vi "Write to the File.vi"(7 "Data Cluster In":T1={"UI Reference"={"All Ctrl's Label's"=[], "ChannelListTree"=refnum, "All Object Ref"=[]}, "Tree Selection"={"Selected Channel"="", "Selected Interface"="", "Selected HW"="", "Tree Root Name"="", "Selected Module"=""}, "Selected File Path"=path "", "Selected HW"={"Slctd Hw Name"=[], "Slctd HW IP"=[]}, "Channel Config Path"=path "", "Interface Data"={"DO Channel's"=[]}, "General Info's"={"Idnentification name"=""}, "Status"="", "Channel Type's"={"Channel Type"=enum."Voltage", "Sub-Type"=enum."Pressure"}, "This VI"=refnum, "Hardware Information "=variant(variant[] [])}, 8 "error in":errorcluster) -> (0 "error out":errorcluster, 5 "Data Cluster Out":T1={"UI Reference"={"All Ctrl's Label's"=[], "ChannelListTree"=refnum, "All Object Ref"=[]}, "Tree Selection"={"Selected Channel"="", "Selected Interface"="", "Selected HW"="", "Tree Root Name"="", "Selected Module"=""}, "Selected File Path"=path "", "Selected HW"={"Slctd Hw Name"=[], "Slctd HW IP"=[]}, "Channel Config Path"=path "", "Interface Data"={"DO Channel's"=[]}, "General Info's"={"Idnentification name"=""}, "Status"="", "Channel Type's"={"Channel Type"=enum."Voltage", "Sub-Type"=enum."Pressure"}, "This VI"=refnum, "Hardware Information "=variant(variant[] [])})   [LabVIEW 2021, in "Configuration.lvlib"]
doc: "<b>Note:</b> This VI was modified by the <b>Validate DQMH Module</b> tool to turn off automatic error handling."
uses:
  Configuration.lvlib
  Module Data--cluster.ctl
  Host-Control's/Configuration UI Reference.ctl
  DO Channel's.ctl
  Config-Channel Type.ctl
  Channel Sub-Type.ctl
  All Interface Data.ctl
  Analog Input Single Channel Data--Cluster.ctl
  Analog Output/Controls/AO Timing Cluster.ctl
  <vilib>/Utility/xml.llb/Read From XML File.vi
  <vilib>/Utility/xml.llb/Read From XML File(string).vi
  <vilib>/Utility/xml.llb/Write to XML File.vi
  <vilib>/Utility/xml.llb/Write to XML File(string).vi
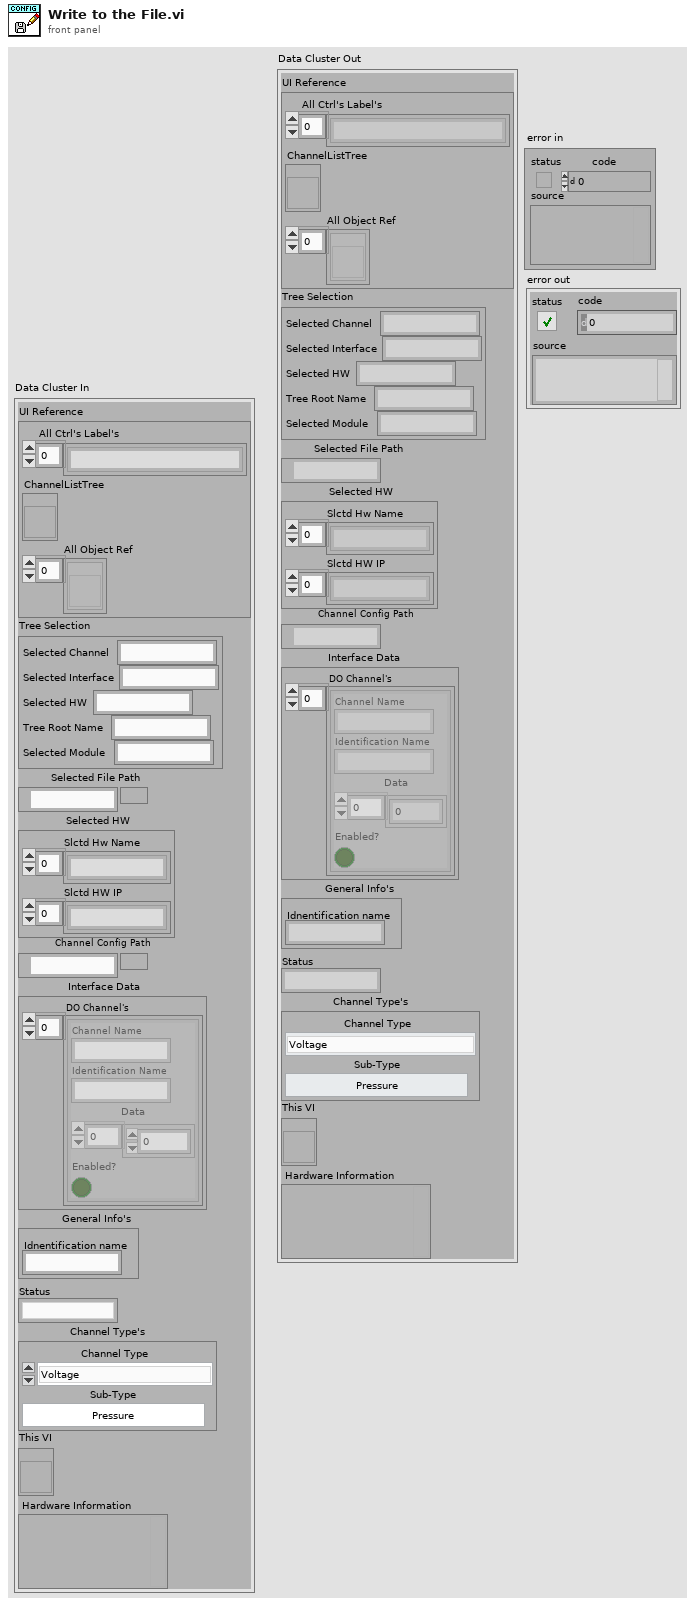
[diagram p1: front panel]
types:
  T1 = typedef "Configuration.lvlib/Module Data--cluster.ctl" = cluster{"UI Reference":T2, "Tree Selection":cluster{"Selected Channel":string, "Selected Interface":string, "Selected HW":string, "Tree Root Name":string, "Selected Module":string}, "Selected File Path":path, "Selected HW":cluster{"Slctd Hw Name":string[], "Slctd HW IP":string[]}, "Channel Config Path":path, "Interface Data":cluster{"DO Channel's":T3}, "General Info's":cluster{"Idnentification name":string}, "Status":string, "Channel Type's":cluster{"Channel Type":T4, "Sub-Type":T5}, "This VI":refnum<vi>, "Hardware Information ":variant}
  T2 = typedef "Configuration UI Reference.ctl" = cluster{"All Ctrl's Label's":string[], "ChannelListTree":refnum<vi>, "All Object Ref":refnum<vi>[]}
  T3 = typedef "Configuration.lvlib/DO Channel's.ctl" = cluster{"Channel Name":string, "Identification Name":string, "Data":u8[], "Enabled?":bool}[]
  T4 = typedef "Configuration.lvlib/Config-Channel Type.ctl" = enum16{"Voltage", "Current", "Thermocouple", "Acclerometer"}
  T5 = typedef "Configuration.lvlib/Channel Sub-Type.ctl" = enum16{"None", "Pressure", "Force"}
  T6 = typedef "Configuration.lvlib/All Interface Data.ctl" = cluster{"DI Config Data":T3, "DO Config Data":T3, "AI Config Data's":cluster{"Module Name":string, "AI Channel's Data":T7[], "Analog Input Timing":T8}[]}
  T7 = typedef "Configuration.lvlib/Analog Input Single Channel Data--Cluster.ctl" = cluster{"Channel Name":string, "Identification Name":string, "Channel Type":T4, "Sub-Type":T5, "Data":string, "Enabled?":bool}
  T8 = typedef "AO Timing Cluster.ctl" = cluster{"samples per channel":i32, "sample mode":i32, "Sampling Rate":dbl}
  T9 = cluster{"Channel Name":string, "Identification Name":string, "Data":u8[], "Enabled?":bool}
  T10 = cluster{"Module Name":string, "AI Channel's Data":T7[], "Analog Input Timing":T8}
  T11 = cluster{"Module Name":string, "AI Channel's Data":T7[], "Analog Input Timing":T8}[]
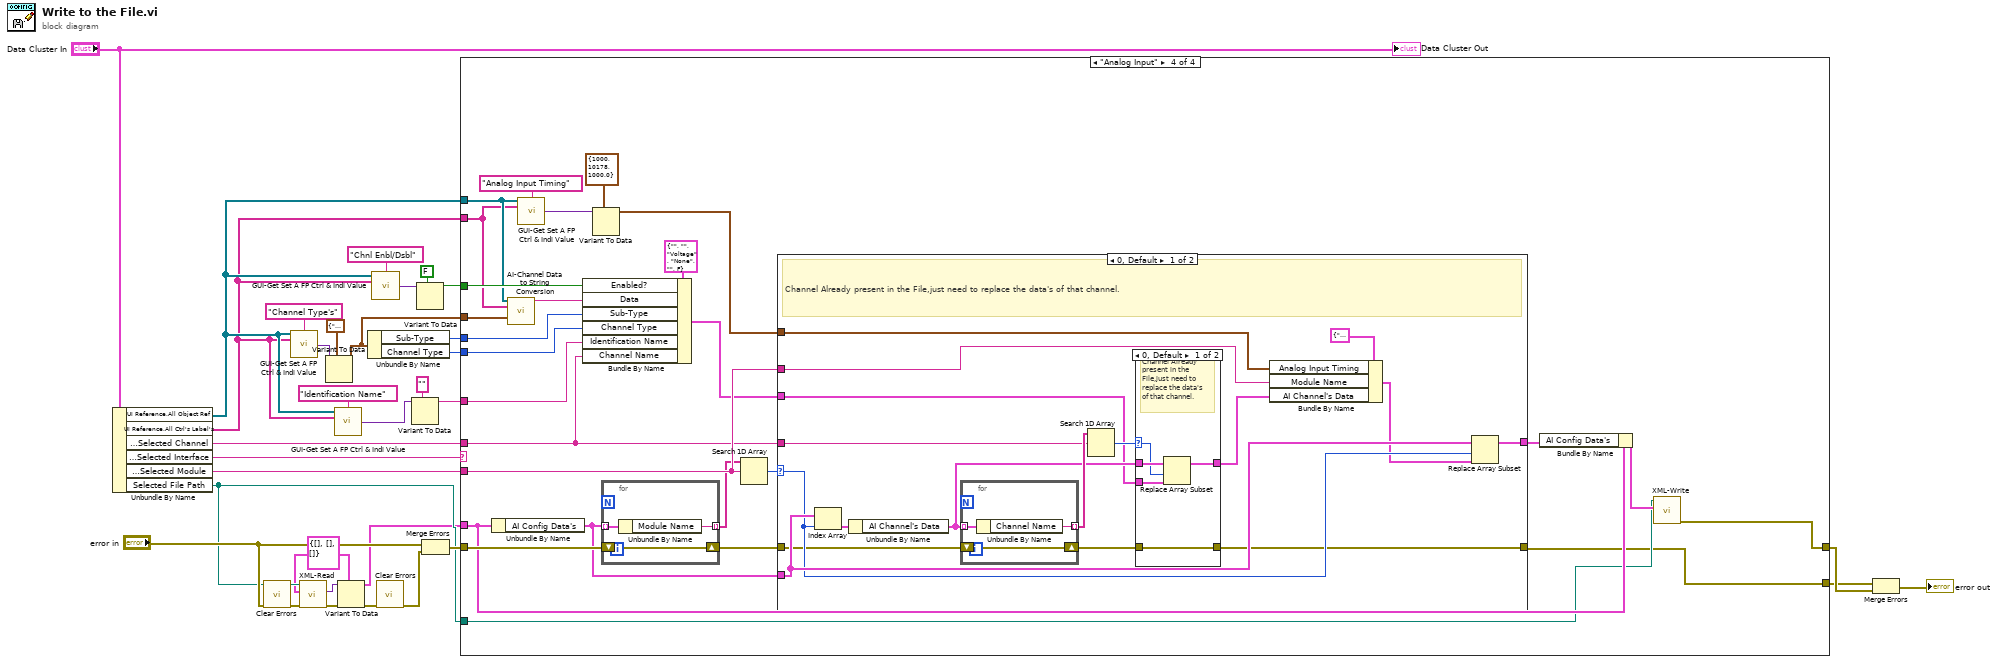
[diagram p0: block diagram]
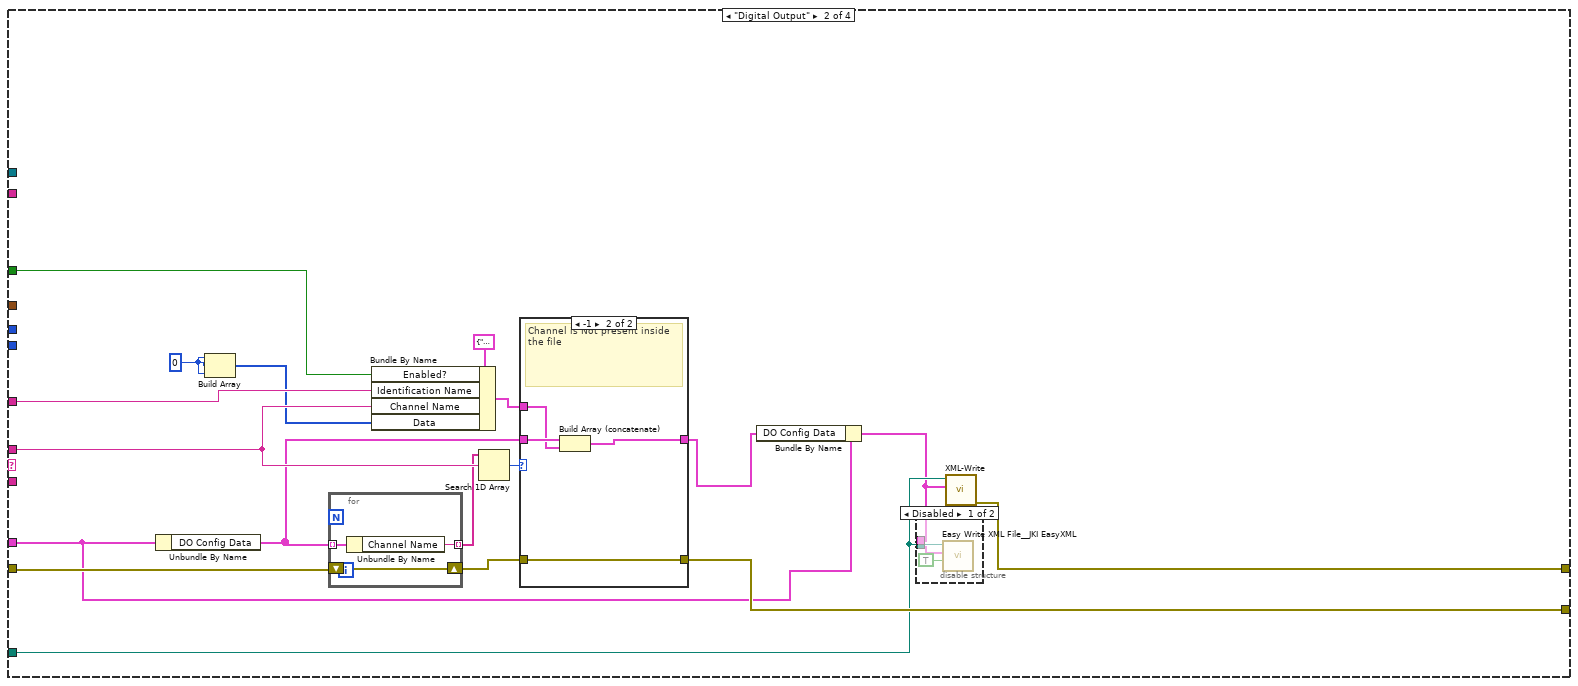
[diagram p3: hidden frame]
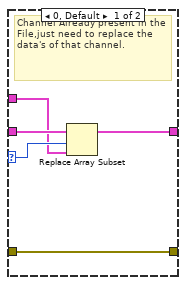
[diagram p5: hidden frame]
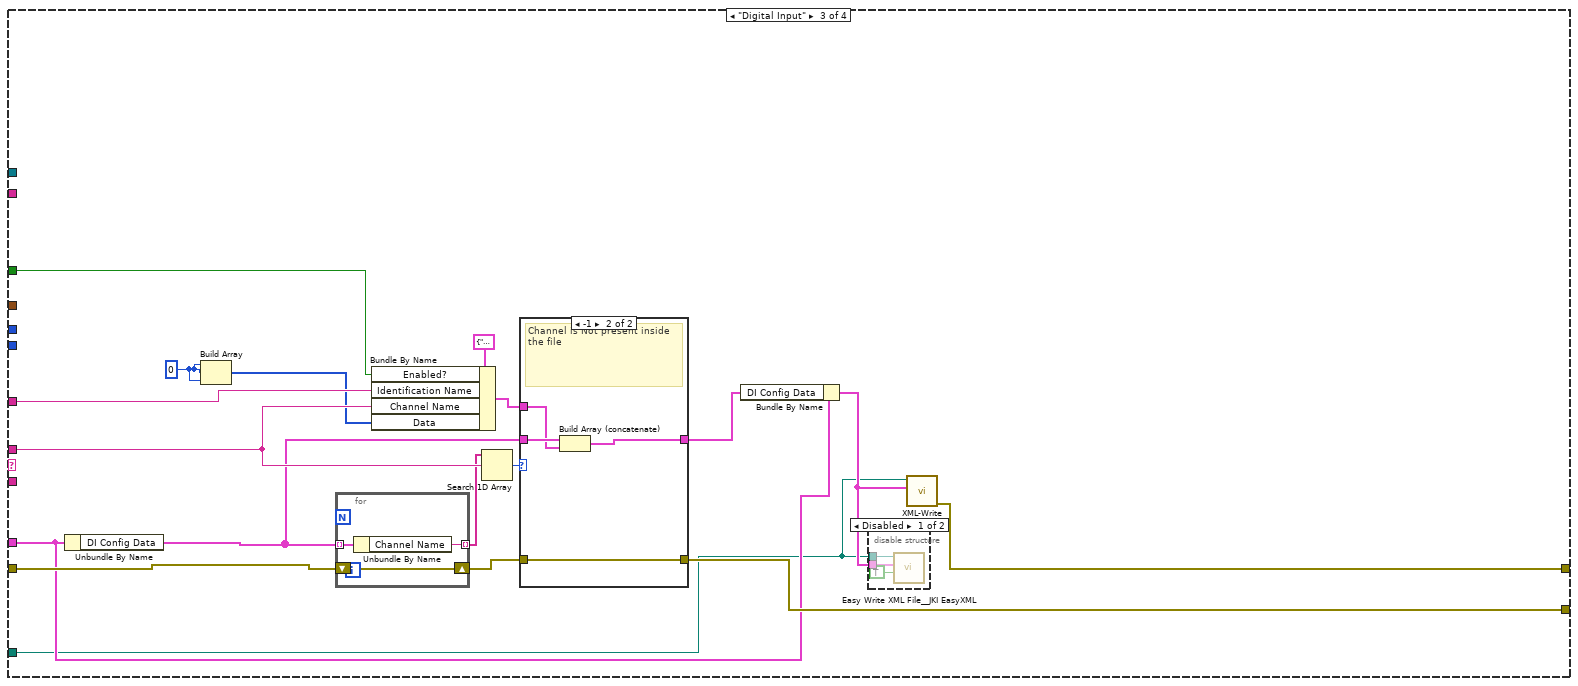
[diagram p6: hidden frame]
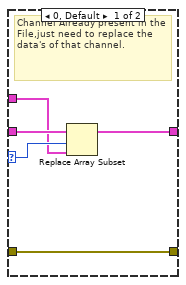
[diagram p8: hidden frame]
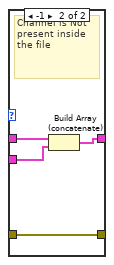
[diagram p9: hidden frame]
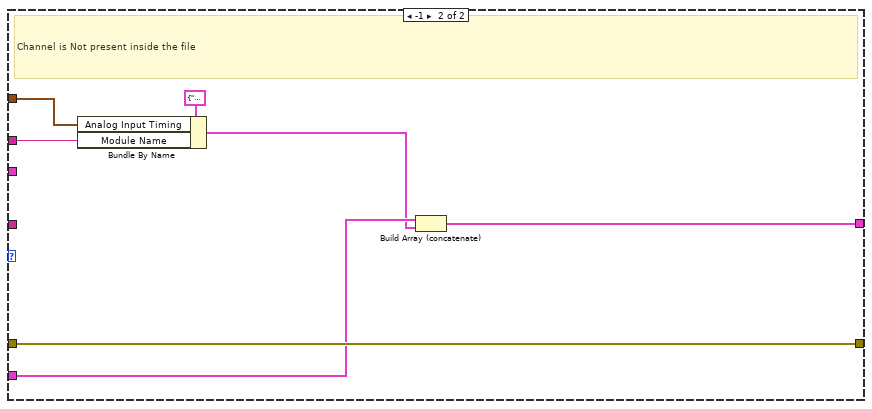
[diagram p10: hidden frame]
diagram:
  w6 = T6 {"DI Config Data"=[], "DO Config Data"=[], "AI Config Data's"=[]} ("Interface Data")
  n1 = Unbundle By Name("Data Cluster In") -> ("UI Reference.All Object Ref"=w10:refnum<vi>[], "UI Reference.All Ctrl's Label's"=w9:string[], "Tree Selection.Selected Channel"=w31:string, "Tree Selection.Selected Interface"=w33:string, "Tree Selection.Selected Module"=w1:string, "Selected File Path"=w8:path)
  n2 = call <vilib>:"Clear Errors.vi"("error in (no error)"="error in") -> ("error out"=w4:errorcluster)  [unwired: 5 in, 1 out]
  n3 = call "GUI-Get Set A FP Ctrl & Indi Value.vi"("All Object Ref"=w10, "Label"="Channel Type's" ("Label In"), "All Object Label"=w9) -> ("Ctrl Value Out"=w15:variant)  [unwired: 9 in, 3 out]
  n4 = call "XML-Read.vi"("error in (no error)"=w4, "Data"=w6, "XML File Path"=w8) -> ("error out"=w3:errorcluster, "Data Out"=w7:variant)  [unwired: 6 in, 1 out]
  n5 = Variant To Data(type=cluster{"Channel Type":T4, "Sub-Type":T5} {"Channel Type"=enum."Voltage", "Sub-Type"=enum."None"} ("Value"), Variant=w15) -> (data=w19:cluster{"Channel Type":T4, "Sub-Type":T5})  [unwired: 1 in, 1 out]
  n6 = call "GUI-Get Set A FP Ctrl & Indi Value.vi"("All Object Ref"=w10, "Label"="Identification Name" ("Label In"), "All Object Label"=w9) -> ("Ctrl Value Out"=w11:variant)  [unwired: 9 in, 3 out]
  n7 = Variant To Data(error in=w3, type=w6, Variant=w7) -> (data=w5:T6, error out=w2:errorcluster)
  n8 = Unbundle By Name(w19) -> ("Sub-Type"=w23:T5, "Channel Type"=w24:T4)
  n9 = call "GUI-Get Set A FP Ctrl & Indi Value.vi"("All Object Ref"=w10, "Label"="Chnl Enbl/Dsbl" ("Label In"), "All Object Label"=w9) -> ("Ctrl Value Out"=w13:variant)  [unwired: 9 in, 3 out]
  n10 = call <vilib>:"Clear Errors.vi"("error in (no error)"=w2) -> ("error out"=w26:errorcluster)  [unwired: 5 in, 1 out]
  n11 = Variant To Data(type="", Variant=w11) -> (data=w21:string)  [unwired: 1 in, 1 out]
  n12 = Variant To Data(type=FALSE, Variant=w13) -> (data=w17:bool)  [unwired: 1 in, 1 out]
  n13 = Merge Errors("error in", w26) -> (w27:errorcluster)
  n14 = case shown="\"Analog Input\"" w33 {
    tunnel: w27 -> [w34 w41 w74 w125]
    tunnel: [w34 w35 w68 w111] -> w29
    tunnel: w31 -> [_ w52 w85 w101]
    tunnel: w21 -> [_ w51 w84 w127]
    tunnel: w5 -> [_ w40 w73 w124]
    tunnel: [w34 w43 w76 w102] -> w28
    tunnel: w8 -> [_ w37 w69 w112]
    tunnel: w24 -> [_ _ _ w123]
    tunnel: w23 -> [_ _ _ w122]
    tunnel: w19 -> [_ _ _ w120]
    tunnel: w17 -> [_ w38 w71 w118]
    tunnel: w10 -> [_ _ _ w115]
    tunnel: w9 -> [_ _ _ w114]
    tunnel: w1 -> [_ _ _ w107]
    frame Default {
    }
    frame "Digital Output" {
      w44 = u8 0 ("Numeric")
      n15 = Unbundle By Name(w40) -> ("DO Config Data"=w42:T3)
      n16 = Build Array(w44, w44, w44) -> (w45:u8[])
      n17 = for {
        tunnel: w42 -> [w66] mode=indexing
        shift-right: [w67] -> w48
        shift-left: w41 -> [w67]
        tunnel: [w65] -> w50 mode=indexing
        n18 = Unbundle By Name(w66) -> ("Channel Name"=w65:string)
      }
      n19 = Bundle By Name(cluster=T9 {"Channel Name"="", "Identification Name"="", "Data"=[], "Enabled?"=FALSE} ("DI Channel's"), "Enabled?"=w38, "Identification Name"=w51, "Channel Name"=w52, "Data"=w45) -> (w47:T9)
      n20 = Search 1D Array(1D array=w50, element=w52) -> (index of element=w49:i32)  [unwired: 1 in]
      n21 = case shown="-1" w49 {
        selector: w49 -> [w58 _]
        tunnel: w48 -> [w60 w64]
        tunnel: [w60 w64] -> w43
        tunnel: w42 -> [w59 w63]
        tunnel: [w57 w62] -> w39
        tunnel: w47 -> [w56 w61]
        frame 0, Default {
          # "Channel Already present in the File,just need to replace the data's of that channel."
          n22 = Replace Array Subset(array=w59, new element=w56, index=w58) -> (w57:T3)
        }
        frame -1 {
          # "Channel is Not present inside the file"
          n23 = Build Array (concatenate)(w63, w61) -> (w62:T3)
        }
      }
      n24 = Bundle By Name(cluster=w40, "DO Config Data"=w39) -> (w36:T6)
      n25 = disable-structure shown="Disabled" {
        disable-tunnel: w37 -> [w54 _]
        disable-tunnel: w36 -> [w53 _]
        frame Disabled {
          n26 = call <vilib>:"Easy Write XML File__JKI EasyXML.vi"("Overwrite File? (false)"=TRUE, "LabVIEW Data"=w53, "XML File Path"=w54) -> ()  [unwired: 7 in, 2 out]
        }
        frame Enabled {
        }
      }
      n27 = call "XML-Write.vi"("Data"=w36, "XML File Path"=w37) -> ("error out"=w35:errorcluster)  [unwired: 7 in, 2 out]
    }
    frame "Digital Input" {
      w77 = u8 0 ("Numeric")
      n28 = Unbundle By Name(w73) -> ("DI Config Data"=w75:T3)
      n29 = Build Array(w77, w77, w77) -> (w78:u8[])
      n30 = for {
        tunnel: w75 -> [w99] mode=indexing
        shift-right: [w100] -> w81
        shift-left: w74 -> [w100]
        tunnel: [w98] -> w83 mode=indexing
        n31 = Unbundle By Name(w99) -> ("Channel Name"=w98:string)
      }
      n32 = Bundle By Name(cluster=T9 {"Channel Name"="", "Identification Name"="", "Data"=[], "Enabled?"=FALSE} ("DI Channel's"), "Enabled?"=w71, "Identification Name"=w84, "Channel Name"=w85, "Data"=w78) -> (w80:T9)
      n33 = Search 1D Array(1D array=w83, element=w85) -> (index of element=w82:i32)  [unwired: 1 in]
      n34 = case shown="-1" w82 {
        selector: w82 -> [w91 _]
        tunnel: w81 -> [w93 w97]
        tunnel: [w93 w97] -> w76
        tunnel: w75 -> [w92 w96]
        tunnel: [w90 w95] -> w72
        tunnel: w80 -> [w89 w94]
        frame 0, Default {
          # "Channel Already present in the File,just need to replace the data's of that channel."
          n35 = Replace Array Subset(array=w92, new element=w89, index=w91) -> (w90:T3)
        }
        frame -1 {
          # "Channel is Not present inside the file"
          n36 = Build Array (concatenate)(w96, w94) -> (w95:T3)
        }
      }
      n37 = Bundle By Name(cluster=w73, "DI Config Data"=w72) -> (w70:T6)
      n38 = disable-structure shown="Disabled" {
        disable-tunnel: w70 -> [w87 _]
        disable-tunnel: w69 -> [w86 _]
        frame Disabled {
          n39 = call <vilib>:"Easy Write XML File__JKI EasyXML.vi"("Overwrite File? (false)"=TRUE, "LabVIEW Data"=w87, "XML File Path"=w86) -> ()  [unwired: 7 in, 2 out]
        }
        frame Enabled {
        }
      }
      n40 = call "XML-Write.vi"("Data"=w70, "XML File Path"=w69) -> ("error out"=w68:errorcluster)  [unwired: 7 in, 2 out]
    }
    frame "Analog Input" {
      n41 = Unbundle By Name(w124) -> ("AI Config Data's"=w108:T11)
      n42 = call "AI-Channel Data to String Conversion.vi"("All Object Ref"=w115, "All Object Label"=w114, "Channel Types'"=w120) -> ("XML String Out"=w121:string)  [unwired: 12 in]
      n43 = call "GUI-Get Set A FP Ctrl & Indi Value.vi"("All Object Ref"=w115, "Label"="Analog Input Timing" ("Label In"), "All Object Label"=w114) -> ("Ctrl Value Out"=w116:variant)  [unwired: 9 in, 3 out]
      n44 = Bundle By Name(cluster=T7 {"Channel Name"="", "Identification Name"="", "Channel Type"=enum."Voltage", "Sub-Type"=enum."None", "Data"="", "Enabled?"=FALSE} ("AI Single Channel Data"), "Enabled?"=w118, "Data"=w121, "Sub-Type"=w122, "Channel Type"=w123, "Identification Name"=w127, "Channel Name"=w101) -> (w105:T7)
      n45 = Variant To Data(type=T8 {"samples per channel"=1000, "sample mode"=10178, "Sampling Rate"=1000.0} ("Analog Input Timing"), Variant=w116) -> (data=w104:T8)  [unwired: 1 in, 1 out]
      n46 = for {
        tunnel: w108 -> [w165] mode=indexing
        shift-right: [w166] -> w110
        shift-left: w125 -> [w166]
        tunnel: [w164] -> w106 mode=indexing
        n47 = Unbundle By Name(w165) -> ("Module Name"=w164:string)
      }
      n48 = Search 1D Array(1D array=w106, element=w107) -> (index of element=w109:i32)  [unwired: 1 in]
      n49 = case shown="0, Default" w109 {
        selector: w109 -> [w141 _]
        tunnel: w110 -> [w139 w163]
        tunnel: [w128 w163] -> w102
        tunnel: w108 -> [w142 w158]
        tunnel: [w144 w162] -> w103
        tunnel: w107 -> [w131 w159]
        tunnel: w101 -> [w137 _]
        tunnel: w105 -> [w133 _]
        tunnel: w104 -> [w130 w160]
        frame 0, Default {
          # "Channel Already present in the File,just need to replace the data's of that channel."
          n50 = Index Array(array=w142, index=w141) -> (element=w140:T10)
          n51 = Unbundle By Name(w140) -> ("AI Channel's Data"=w135:T7[])
          n52 = for {
            tunnel: w135 -> [w155] mode=indexing
            shift-right: [w156] -> w134
            shift-left: w139 -> [w156]
            tunnel: [w154] -> w138 mode=indexing
            n53 = Unbundle By Name(w155) -> ("Channel Name"=w154:string)
          }
          n54 = Search 1D Array(1D array=w138, element=w137) -> (index of element=w136:i32)  [unwired: 1 in]
          n55 = case shown="0, Default" w136 {
            selector: w136 -> [w147 _]
            tunnel: w134 -> [w149 w153]
            tunnel: [w149 w153] -> w128
            tunnel: w135 -> [w148 w152]
            tunnel: [w146 w151] -> w132
            tunnel: w133 -> [w145 w150]
            frame 0, Default {
              # "Channel Already present in the File,just need to replace the data's of that channel."
              n56 = Replace Array Subset(array=w148, new element=w145, index=w147) -> (w146:T7[])
            }
            frame -1 {
              # "Channel is Not present inside the file"
              n57 = Build Array (concatenate)(w152, w150) -> (w151:T7[])
            }
          }
          n58 = Bundle By Name(cluster=T10 {"Module Name"="", "AI Channel's Data"=[], "Analog Input Timing"={"samples per channel"=0, "sample mode"=0, "Sampling Rate"=0.0}} ("AI Config Data's"), "Analog Input Timing"=w130, "Module Name"=w131, "AI Channel's Data"=w132) -> (w129:T10)
          n59 = Replace Array Subset(array=w142, new element=w129, index=w141) -> (w144:T11)
        }
        frame -1 {
          # "Channel is Not present inside the file"
          n60 = Bundle By Name(cluster=T10 {"Module Name"="", "AI Channel's Data"=[], "Analog Input Timing"={"samples per channel"=0, "sample mode"=0, "Sampling Rate"=0.0}} ("AI Config Data's"), "Analog Input Timing"=w160, "Module Name"=w159) -> (w157:T10)
          n61 = Build Array (concatenate)(w158, w157) -> (w162:T11)
        }
      }
      n62 = Bundle By Name(cluster=w124, "AI Config Data's"=w103) -> (w113:T6)
      n63 = call "XML-Write.vi"("Data"=w113, "XML File Path"=w112) -> ("error out"=w111:errorcluster)  [unwired: 7 in, 2 out]
    }
  }
  n64 = Merge Errors(w28, w29) -> (→"error out":errorcluster)
  "Data Cluster Out" <- "Data Cluster In"
